vi "pulse_shaping.vi"(8 "error in (no error)":errorcluster, 10 "input":cdb[](array[numeric]), 11 "Modulation Parameters In":T1={"TX Parameters"={"TX Oversample Factor"=4, "TX Sample Rate"=0.0}, "TX/RX Shared Parameters"={"Modulation Type"=enum."OOK", "Packet Length"=128, "# of Iterations"=0.0, "Pulse Shaping Parameters"={"Pulse Shaping Filter"=enum."none", "Filter Length (symbols)"=32, "Filter Parameter"=0.8, "modulation type"=enum."FSK"}, "Header/Tail Control Information"={"Training Sequence Type"=enum."", "Zero Pad Length"=0.0}}}) -> (0 "error out":errorcluster, 1 "filter coefficients":dbl[](array[numeric]) format="%.2f", 2 "output":cdb[](array[numeric]), 3 "Modulation Parameters Out":T1={"TX Parameters"={"TX Oversample Factor"=4, "TX Sample Rate"=0.0}, "TX/RX Shared Parameters"={"Modulation Type"=enum."OOK", "Packet Length"=128, "# of Iterations"=0.0, "Pulse Shaping Parameters"={"Pulse Shaping Filter"=enum."none", "Filter Length (symbols)"=32, "Filter Parameter"=0.8, "modulation type"=enum."FSK"}, "Header/Tail Control Information"={"Training Sequence Type"=enum."", "Zero Pad Length"=0.0}}})   [LabVIEW 2012]
uses:
  <vilib>/Analysis/2dsp.llb/Upsample (CDB).vi
  <vilib>/Analysis/2dsp.llb/1D Convolution (CDB).vi
  <vilib>/addons/Modulation/niDMT.lvlib
  <vilib>/Analysis/NI_AALPro.lvlib
panel:
  out "Filter Length (symbols)":i32
  out "Waveform Graph":dbl[](graph)
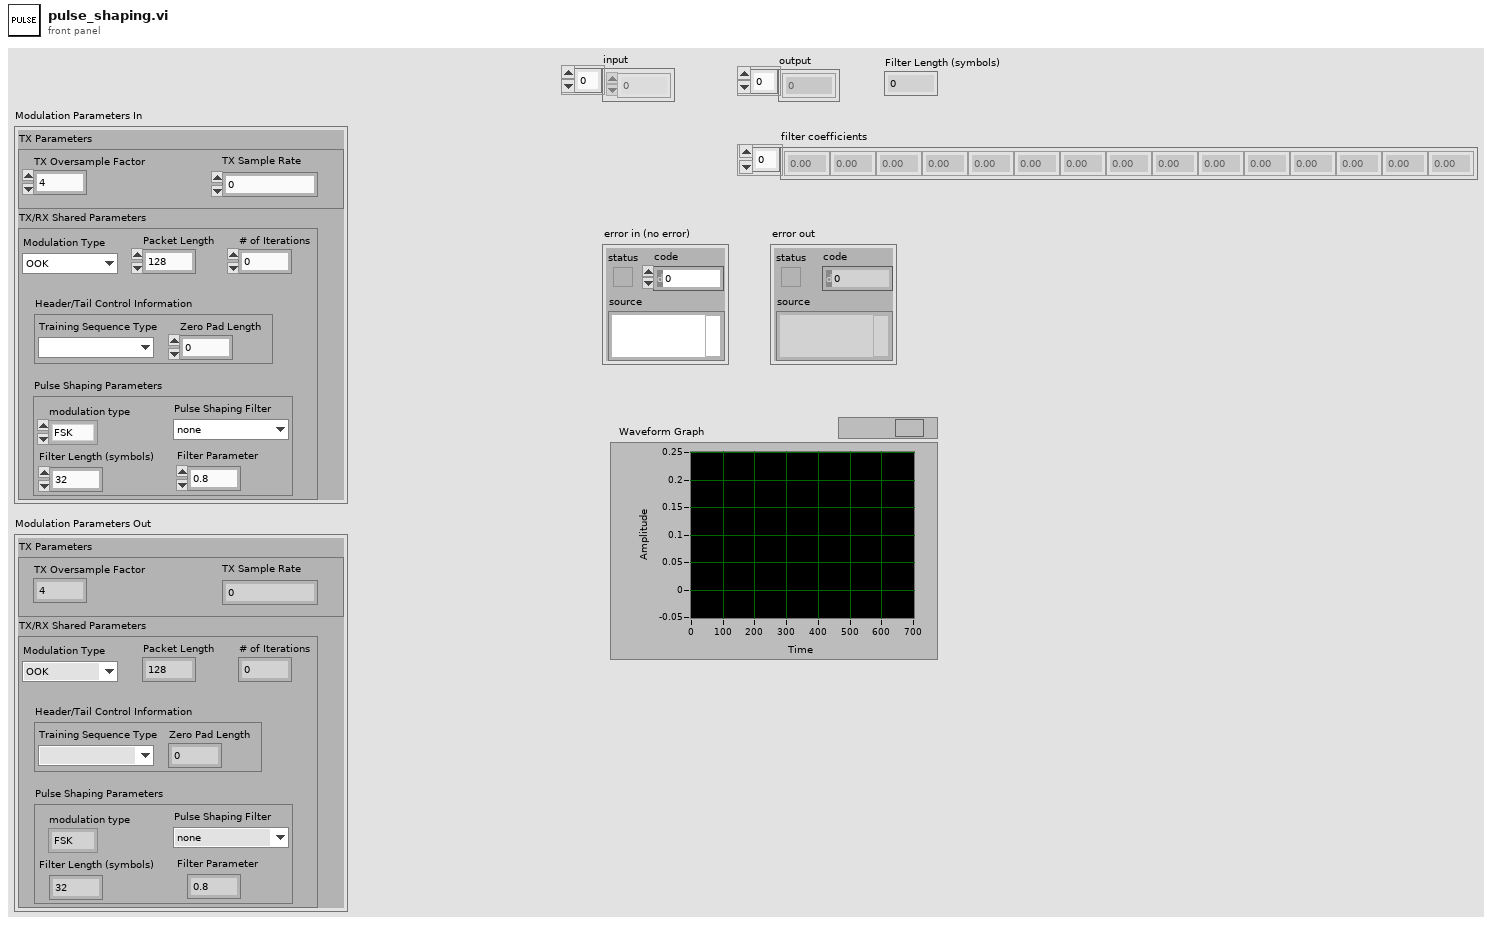
[diagram p1: front panel]
types:
  T1 = cluster{"TX Parameters":cluster{"TX Oversample Factor":i32, "TX Sample Rate":dbl}, "TX/RX Shared Parameters":cluster{"Modulation Type":enum16{"OOK", "FSK"}, "Packet Length":i32, "# of Iterations":dbl, "Pulse Shaping Parameters":cluster{"Pulse Shaping Filter":enum16{"none", "Raised Cosine", "Root Raised Cos", "Gaussian"}, "Filter Length (symbols)":i32, "Filter Parameter":dbl, "modulation type":enum16{"FSK", "PSK", "QAM", "MSK", "PAM", "ASK", "CPM"}}, "Header/Tail Control Information":cluster{"Training Sequence Type":enum16{""}, "Zero Pad Length":dbl}}}
  T2 = cluster{"Pulse Shaping Filter":enum16{"none", "Raised Cosine", "Root Raised Cos", "Gaussian"}, "Filter Length (symbols)":i32, "Filter Parameter":dbl, "modulation type":enum16{"FSK", "PSK", "QAM", "MSK", "PAM", "ASK", "CPM"}}
  T3 = enum16{"FSK", "PSK", "QAM", "MSK", "PAM", "ASK", "CPM"}
  T4 = enum16{"none", "Raised Cosine", "Root Raised Cos", "Gaussian"}
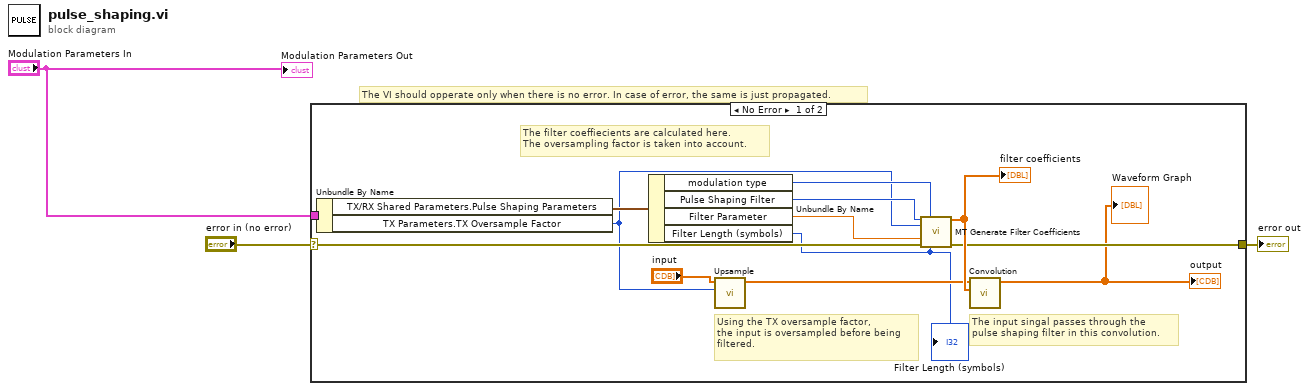
[diagram p0: block diagram]
diagram:
  # "The VI should opperate only when there is no error. In case of error, the same is just propagated."
  n1 = case shown="No Error" "error in (no error)" {
    selector: "error in (no error)" -> [w14 w17]
    tunnel: "Modulation Parameters In" -> [w15 _]
    tunnel: [w10 w17] -> w2
    frame No Error {
      # "The input singal passes through the\npulse shaping filter in this convolution."
      # "The filter coeffiecients are calculated here.\nThe oversampling factor is taken into account."
      # "Using the TX oversample factor,\nthe input is oversampled before being\nfiltered."
      n2 = Unbundle By Name(w15) -> ("TX/RX Shared Parameters.Pulse Shaping Parameters"=w16:T2, "TX Parameters.TX Oversample Factor"=w7:i32)
      n3 = Unbundle By Name(w16) -> ("modulation type"=w9:T3, "Pulse Shaping Filter"=w8:T4, "Filter Parameter"=w6:dbl, "Filter Length (symbols)"=w5:i32)
      "Filter Length (symbols)" <- w5
      n4 = call-poly <vilib>:"Upsample.vi"("upsampling factor"=w7, "X"="input") -> ("Upsampled Array"=w11:cdb[])  [unwired: 8 in, 1 out]
      n5 = call <vilib>:"MT Generate Filter Coefficients.vi"("pulse shaping filter (none)"=w8, "modulation type"=w9, "pulse shaping samples per symbol (16)"=w7, "filter parameter"=w6, "error in (no error)"=w14, "filter length (symbols)"=w5) -> ("pulse shaping filter coefficients"=w13:dbl[], "error out"=w10:errorcluster)  [unwired: 7 in, 1 out]
      "filter coefficients" <- w13
      n6 = call-poly <vilib>:"Convolution.vi"("Y"=w13, "X"=w11) -> ("X * Y"=→"output" →"Waveform Graph":cdb[])  [unwired: 8 in, 1 out]
    }
    frame Error {
    }
  }
  "error out" <- w2
  "Modulation Parameters Out" <- "Modulation Parameters In"
